vi "Pre Launch Init.vi"(11 "Field Drawer in":refnum<class "Field Drawer.lvclass">) -> (0 "error out":errorcluster, 3 "Field Drawer out":refnum<class "Field Drawer.lvclass">)   [LabVIEW 2022 SP3, in "Vision.lvlib" / "Field Drawer.lvlib" / "Field Drawer.lvclass"]
doc: "(<B>Filename</B>: Actor Framework.lvlib:Actor.lvclass:Pre Launch Init.vi)\n\nDefines behavior that occurs after the Launch Actor method is invoked but before the actor's Actor Core method begins running.\n\nThe Pre Launch Init method is guaranteed to finish before the Launch Actor method returns to its caller and before the actor itself receives any messages. Any references that the Pre Launch Init method obtains are guaranteed to have the same lifetime as the actor itself. Any errors that the Pre Launch Init method returns will abort the launch.\n\nBy default, this method does nothing. A descendant class may override it to define behavior."
uses:
  Field Drawer.lvclass
  Field Drawer.lvclass/Field Drawer.ctl
  <vilib>/ActorFramework/Actor/Actor.lvclass
  Old vision/Controls/Field Size.ctl
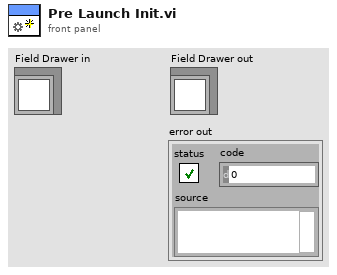
[diagram p1: front panel]
types:
  T1 = typedef "Field Size.ctl" = cluster{"line_width":u32, "field_length":u32, "field_width":u32, "boundary_width":u32, "referee_width":u32, "goal_width":u32, "goal_depth":u32, "goal_wall_width":u32, "center_circle_radius":u32, "defense_radius":u32, "defense_stretch":u32, "free_kick_from_defense_dist":u32, "penalty_spot_from_field_line_dist":u32, "penalty_line_from_spot_dist":u32}
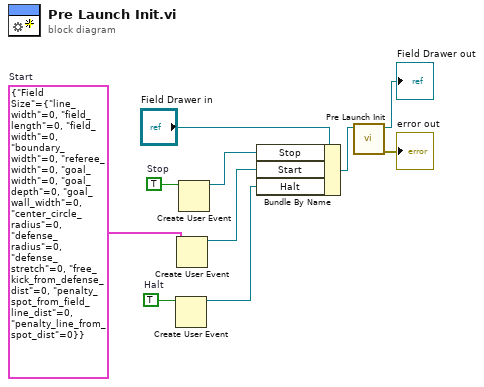
[diagram p0: block diagram]
diagram:
  w1 = cluster{"Field Size":T1} {"Field Size"={"line_width"=0, "field_length"=0, "field_width"=0, "boundary_width"=0, "referee_width"=0, "goal_width"=0, "goal_depth"=0, "goal_wall_width"=0, "center_circle_radius"=0, "defense_radius"=0, "defense_stretch"=0, "free_kick_from_defense_dist"=0, "penalty_spot_from_field_line_dist"=0, "penalty_line_from_spot_dist"=0}}  # Start
  w4 = TRUE  # Halt
  w8 = TRUE  # Stop
  n1 = Create User Event(user event datatype=w4) -> (user event=w2:refnum<user-event>)  [unwired: 1 in, 1 out]
  n2 = Create User Event(user event datatype=w1) -> (user event=w3:refnum<user-event>)  [unwired: 1 in, 1 out]
  n3 = Create User Event(user event datatype=w8) -> (user event=w5:refnum<user-event>)  [unwired: 1 in, 1 out]
  n4 = Bundle By Name(cluster="Field Drawer in", "Stop"=w5, "Start"=w3, "Halt"=w2) -> (w6:refnum<class "Field Drawer.lvclass">)
  n5 = call-parent "Pre Launch Init.vi"("Actor in"=w6) -> ("error out"=→"error out":errorcluster, "Actor out"=→"Field Drawer out":refnum<class "Field Drawer.lvclass">)  [unwired: 9 in]
